vi "myRIOXC Set Pin Info.vi"(7 "Size":i32=34, 9 "Pin Info Array":T2, 10 "Pin ID Map":variant, 11 "Display State In in":T1 caption="State") -> (1 "Data":bool[](array[boolean]), 3 "Display State In out":T1 caption="State")   [LabVIEW 2021]
uses:
  <vilib>/myRIO/Common/Instrument Driver Framework/Utilities/xctls/utilities/typedefs/myRIOXC Pin Info Array.ctl
  <vilib>/myRIO/Common/Instrument Driver Framework/Utilities/xctls/utilities/typedefs/myRIOXC Pin Info.ctl
  <vilib>/myRIO/Common/Instrument Driver Framework/Utilities/xctls/utilities/typedefs/myRIOXC Display State.ctl
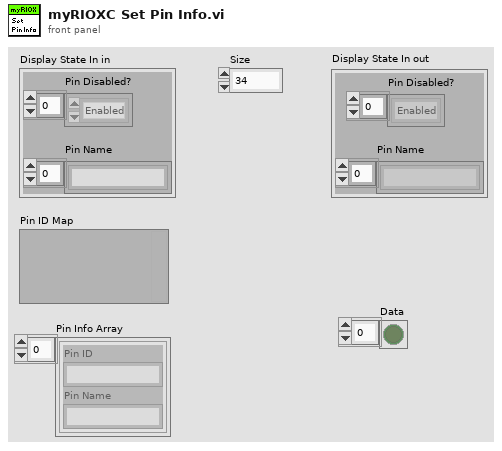
[diagram p1: front panel]
types:
  T1 = typedef "myRIOXC Display State.ctl" = cluster{"Pin Disabled?":enum8{"Enabled", "Disabled", "Disabled and Grayed Out"}[], "Pin Name":string[]}
  T2 = typedef "myRIOXC Pin Info Array.ctl" = T3[]
  T3 = typedef "myRIOXC Pin Info.ctl" = cluster{"Pin ID":string, "Pin Name":string}
  T4 = enum8{"Enabled", "Disabled", "Disabled and Grayed Out"}
  T5 = enum8{"Enabled", "Disabled", "Disabled and Grayed Out"}[]
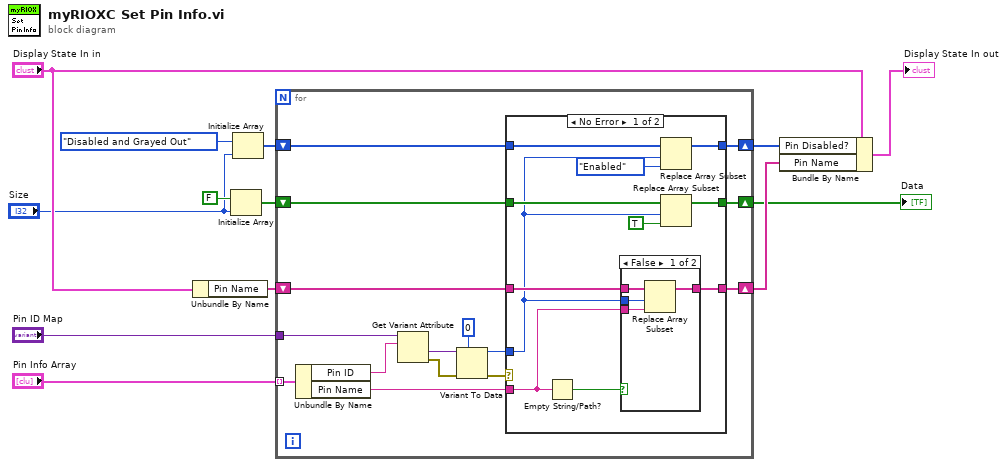
[diagram p0: block diagram]
diagram:
  n1 = Unbundle By Name("Display State In in") -> ("Pin Name"=w10:string[])
  n2 = Initialize Array(FALSE, "Size") -> (w2:bool[])
  n3 = Initialize Array(T4."Disabled and Grayed Out" ("Disabled"), "Size") -> (w8:T5)
  n4 = for {
    tunnel: "Pin Info Array" -> [w28] mode=indexing
    shift-right: [w27] -> w11
    shift-left: w8 -> [w26]
    shift-right: [w25] -> w12
    shift-left: w10 -> [w24]
    tunnel: "Pin ID Map" -> [w22]
    shift-right: [w17] -> w1
    shift-left: w2 -> [w18]
    n5 = Unbundle By Name(w28) -> ("Pin ID"=w23:string, "Pin Name"=w21:string)
    n6 = Get Variant Attribute(Variant=w22, name=w23) -> (value=w20:variant, error out=w15:errorcluster)  [unwired: 2 in, 2 out]
    n7 = Variant To Data(error in=w15, type=0, Variant=w20) -> (data=w16:i32, error out=w14:errorcluster)
    n8 = case shown="No Error" w14 {
      tunnel: [w39 w45] -> w27
      tunnel: w26 -> [w38 w45]
      tunnel: [w37 w47] -> w25
      tunnel: w24 -> [w31 w47]
      tunnel: w21 -> [w36 _]
      tunnel: w18 -> [w34 w46]
      tunnel: [w33 w46] -> w17
      tunnel: w16 -> [w30 _]
      frame No Error {
        n9 = Empty String/Path?(string/path=w36) -> (empty?=w32:bool)
        n10 = case shown="False" w32 {
          tunnel: [w43 w44] -> w37
          tunnel: w31 -> [w42 w44]
          tunnel: w36 -> [w41 _]
          tunnel: w30 -> [w40 _]
          frame False {
            n11 = Replace Array Subset(array=w42, new element=w41, index=w40) -> (w43:string[])
          }
          frame True {
          }
        }
        n12 = Replace Array Subset(array=w38, new element=T4."Enabled" ("Disabled"), index=w30) -> (w39:T5)
        n13 = Replace Array Subset(array=w34, new element=TRUE ("new element/subarray"), index=w30) -> (w33:bool[])
      }
      frame Error {
      }
    }
  }
  "Data" <- w1
  n14 = Bundle By Name(cluster="Display State In in", "Pin Disabled?"=w11, "Pin Name"=w12) -> (→"Display State In out":T1)
